vi "Pre Launch Init.vi"(11 "Lissajous Viewer in":refnum<class "Lissajous Viewer.lvclass">) -> (0 "error out":errorcluster, 3 "Lissajous Viewer out":refnum<class "Lissajous Viewer.lvclass">)   [LabVIEW 2020, in "Lissajous Viewer.lvlib" / "Lissajous Viewer.lvclass"]
doc: "Initializes the panel actor. Creates the Panel Helper.\n\n----\nPlease see the following web address for additional documentation and tutorial information:\nhttp://www.mooregoodideas.com/mgi-panel-manager/\n\nAuthor: Derek Trepanier\n\nCopyright (c) 2018, Moore Good Ideas, Inc.\n\nAll rights reserved.\n\nRedistribution and use in source and binary forms, with or without modification, are permitted provided that the following conditions are met:\n\n * Redistributions of source code must retain the above copyright notice, this list of conditions and the following disclaimer.\n * Redistributions in binary form must reproduce the above copyright notice, this list of conditions and the following disclaimer in the documentation and/or other materials provided with the distribution.\n * Neither the name of Moore Good Ideas, Inc. nor the names of its contributors may be used to endorse or promote products derived from this software without specific prior written permission.\n\nTHIS SOFTWARE IS PROVIDED BY THE COPYRIGHT HOLDERS AND CONTRIBUTORS \"AS IS\" AND ANY EXPRESS OR IMPLIED WARRANTIES, INCLUDING, BUT NOT LIMITED TO, THE IMPLIED WARRANTIES OF MERCHANTABILITY AND FITNESS FOR A PARTICULAR PURPOSE ARE DISCLAIMED. IN NO EVENT SHALL THE COPYRIGHT OWNER OR CONTRIBUTORS BE LIABLE FOR ANY DIRECT, INDIRECT, INCIDENTAL, SPECIAL, EXEMPLARY, OR CONSEQUENTIAL DAMAGES (INCLUDING, BUT NOT LIMITED TO, PROCUREMENT OF SUBSTITUTE GOODS OR SERVICES; LOSS OF USE, DATA, OR PROFITS; OR BUSINESS INTERRUPTION) HOWEVER CAUSED AND ON ANY THEORY OF LIABILITY, WHETHER IN CONTRACT, STRICT LIABILITY, OR TORT (INCLUDING NEGLIGENCE OR OTHERWISE) ARISING IN ANY WAY OUT OF THE USE OF THIS SOFTWARE, EVEN IF ADVISED OF THE POSSIBILITY OF SUCH DAMAGE."
uses:
  Lissajous Viewer.lvclass
  Lissajous Viewer.lvclass/Lissajous Viewer.ctl
  <vilib>/MGI/Panel Manager/Panel Actor/Panel Actor/Panel Actor.lvclass
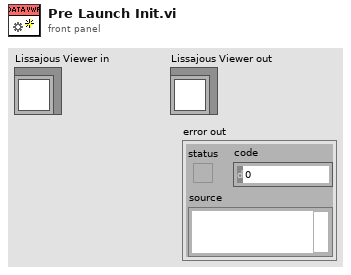
[diagram p1: front panel]
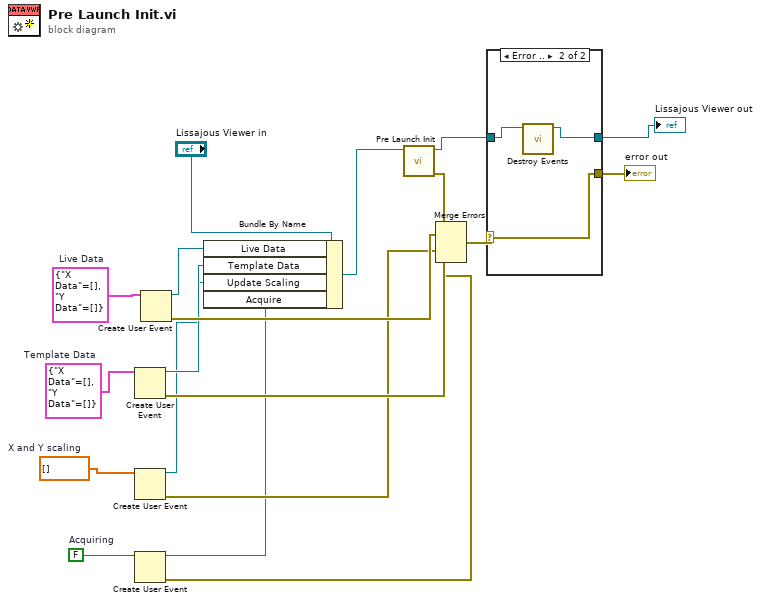
[diagram p0: block diagram]
diagram:
  w3 = FALSE  # Acquiring
  w5 = dbl[] []  # X and Y scaling
  w15 = cluster{"X Data":dbl[], "Y Data":dbl[]} {"X Data"=[], "Y Data"=[]}  # Template Data
  w19 = cluster{"X Data":dbl[], "Y Data":dbl[]} {"X Data"=[], "Y Data"=[]}  # Live Data
  n1 = Create User Event(user event datatype=w15) -> (user event=w10:refnum<user-event>, error out=w14:errorcluster)  [unwired: 1 in]
  n2 = Create User Event(user event datatype=w5) -> (user event=w4:refnum<user-event>, error out=w6:errorcluster)  [unwired: 1 in]
  n3 = Create User Event(user event datatype=w3) -> (user event=w1:refnum<user-event>, error out=w2:errorcluster)  [unwired: 1 in]
  n4 = Create User Event(user event datatype=w19) -> (user event=w11:refnum<user-event>, error out=w16:errorcluster)  [unwired: 1 in]
  n5 = Bundle By Name(cluster="Lissajous Viewer in", "Live Data"=w11, "Template Data"=w10, "Update Scaling"=w4, "Acquire"=w1) -> (w12:refnum<class "Lissajous Viewer.lvclass">)
  n6 = call-parent "Pre Launch Init.vi"("Panel Actor in"=w12) -> ("error out"=w17:errorcluster, "Panel Actor out"=w8:refnum<class "Lissajous Viewer.lvclass">)  [unwired: 9 in]
  n7 = Merge Errors(w17, w16, w14, w6, w2) -> (w9:errorcluster)
  n8 = case shown="Error .." w9 {
    selector: w9 -> [w21 w24]
    tunnel: [w21 w24] -> w18
    tunnel: [w20 w22] -> w7
    tunnel: w8 -> [w20 w23]
    frame No Error {
    }
    frame Error {
      n9 = call "Destroy Events.vi"("Lissajous Viewer in"=w23) -> ("Lissajous Viewer out"=w22:refnum<class "Lissajous Viewer.lvclass">)  [unwired: 9 in, 1 out]
    }
  }
  "error out" <- w18
  "Lissajous Viewer out" <- w7
